vi "Shooter RPM Calc.vi"(7 "Backspin":dbl=400.0, 8 "Height Trim":dbl, 9 "Distance Trim":dbl, 10 "Height":dbl, 11 "Distance":dbl) -> (1 "ok":bool, 2 "Bottom RPM":dbl, 3 "Top RPM":dbl)   [LabVIEW 2011]
panel:
  out "Raw RPM":dbl
  out "Scaled H":dbl
  out "SF":dbl
  out "xmax":dbl
  out "k":dbl
  out "a":dbl
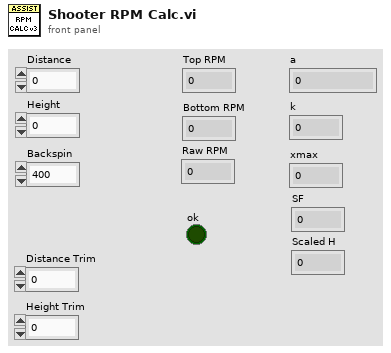
[diagram p1: front panel]
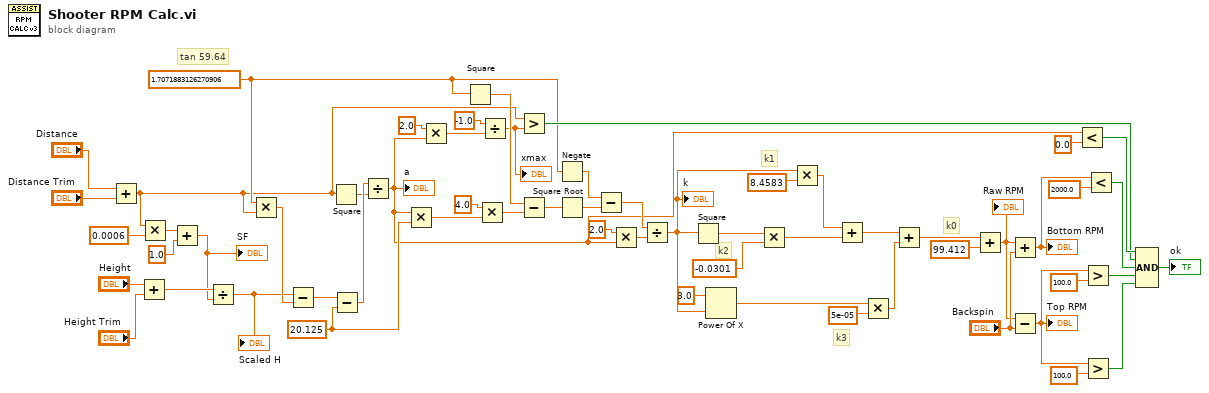
[diagram p0: block diagram]
diagram:
  w14 = 1.7071883126270906 ("x")
  w53 = 20.125 ("y")
  # "k0"
  # "k3"
  # "k2"
  # "k1"
  # "tan 59.64"
  n1 = Add(x="Distance", y="Distance Trim") -> (x+y=w8:dbl)
  n2 = Add(x="Height", y="Height Trim") -> (x+y=w4:dbl)
  n3 = Multiply(x=w8, y=0.0006) -> (x*y=w6:dbl)
  n4 = Add(x=w6, y=1.0) -> (x+y=w3:dbl)
  "SF" <- w3
  n5 = Divide(x=w4, y=w3) -> (x/y=w2:dbl)
  "Scaled H" <- w2
  n6 = Multiply(x=w14, y=w8) -> (x*y=w59:dbl)
  n7 = Subtract(x=w2, y=w59) -> (x-y=w58:dbl)
  n8 = Square(x=w8) -> (x^2=w56:dbl)
  n9 = Subtract(x=w58, y=w53) -> (x-y=w57:dbl)
  n10 = Divide(x=w57, y=w56) -> (x/y=w29:dbl)
  "a" <- w29
  n11 = Multiply(x=w29, y=w53) -> (x*y=w52:dbl)
  n12 = Multiply(x=2.0, y=w29) -> (x*y=w28:dbl)
  n13 = Square(x=w14) -> (x^2=w54:dbl)
  n14 = Multiply(x=4.0, y=w52) -> (x*y=w50:dbl)
  n15 = Divide(x=-1.0, y=w28) -> (x/y=w26:dbl)
  "xmax" <- w26
  n16 = Greater?(x=w8, y=w26) -> (0:w25:bool)
  n17 = Subtract(x=w54, y=w50) -> (x-y=w49:dbl)
  n18 = Negate(x=w14) -> (-x=w55:dbl)
  n19 = Square Root(x=w49) -> (sqrt(x)=w48:dbl)
  n20 = Subtract(x=w55, y=w48) -> (x-y=w46:dbl)
  n21 = Multiply(x=2.0, y=w29) -> (x*y=w45:dbl)
  n22 = Divide(x=w46, y=w45) -> (x/y=w33:dbl)
  "k" <- w33
  n23 = Square(x=w33) -> (x^2=w43:dbl)
  n24 = Power Of X(1:w33, 2:3.0 ("y")) -> (0:w37:dbl)
  n25 = Multiply(x=w43, y=-0.0301) -> (x*y=w41:dbl)
  n26 = Multiply(x=w33, y=8.4583) -> (x*y=w42:dbl)
  n27 = Add(x=w42, y=w41) -> (x+y=w40:dbl)
  n28 = Multiply(x=w37, y=5e-05) -> (x*y=w35:dbl)
  n29 = Add(x=w40, y=w35) -> (x+y=w39:dbl)
  n30 = Add(x=w39, y=99.412) -> (x+y=w22:dbl)
  "Raw RPM" <- w22
  n31 = Add(x=w22, y="Backspin") -> (x+y=w21:dbl)
  "Bottom RPM" <- w21
  n32 = Subtract(x=w22, y="Backspin") -> (x-y=w11:dbl)
  "Top RPM" <- w11
  n33 = Less?(x=w29, y=0.0) -> (x < y?=w31:bool)
  n34 = Greater?(x=w11, y=100.0) -> (0:w12:bool)
  n35 = Greater?(x=w11, y=100.0) -> (0:w9:bool)
  n36 = Less?(x=w21, y=2000.0) -> (x < y?=w24:bool)
  n37 = Compound Arithmetic op=AND(w31, w25, w24, w12, w9) -> (→"ok":bool)
